vi "WriteTree.vi"(8 "error in":errorcluster, 11 "cRIO repo in":refnum<class "database file.lvclass">) -> (0 "error out":errorcluster, 2 "root":T1, 3 "repository out":refnum<class "NISE_CEF_Repository.lvclass">)   [LabVIEW 2013, in "database file.lvclass"]
uses:
  database file.lvclass
  <vilib>/NI/Configuration Framework/Repository/NISE_CEF_Repository.lvclass
  <vilib>/NI/Configuration Framework/Node/NodeRef.ctl
  <vilib>/NI/Configuration Framework/Node/NISE_CEF_Node.lvclass
  can port/can port.lvclass
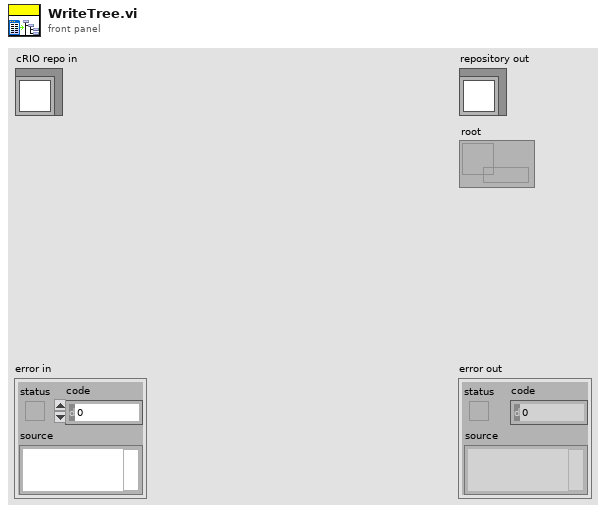
[diagram p1: front panel]
types:
  T1 = typedef "NISE_CEF_Node.lvclass/NodeRef.ctl" = refnum<data-value>
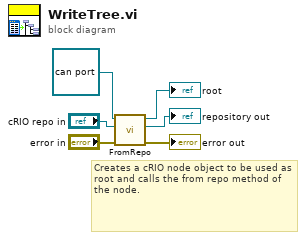
[diagram p0: block diagram]
diagram:
  # "Creates a cRIO node object to be used as root and calls the from repo method of the node."
  n1 = call-dynamic "FromRepo.vi"("error in"="error in", "repository in"="cRIO repo in", "cRIO in"=refnum<class "can port.lvclass"> refnum ("cRIO.lvclass")) -> ("error out"=→"error out":errorcluster, "repository out"=→"repository out":refnum<class "NISE_CEF_Repository.lvclass">, "node"=→"root":T1)  [unwired: 6 in]
